vi "FWHM-TIME.vi"() -> ()   [LabVIEW 2014]
doc: "André Romero - 2017\nandretec@ifsc.usp.br"
uses:
  <vilib>/Utility/file.llb/Write To Spreadsheet File (DBL).vi
panel:
  out "Seconds":i32
  in  "Average":i32=1
  out "Waveform Graph":dbl[](graph)
  out "FWHM":dbl=7.6633162264068915
  in  "stop":bool
  out "XY Graph":T1(graph)
  in  "Correct Electrical Dark":bool=TRUE
  in  "Integration Time (ms)":i32=100
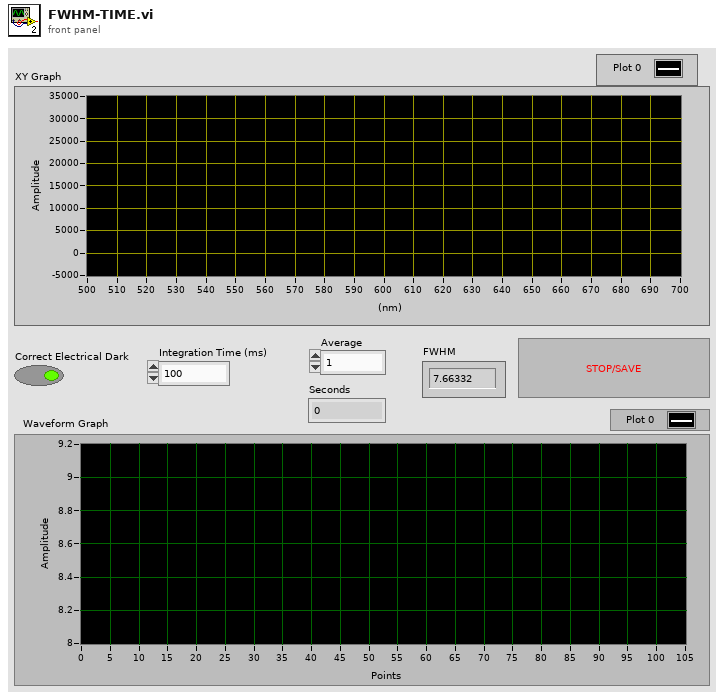
[diagram p1: front panel]
types:
  T1 = cluster{"WL Values":dbl[], "Spectrum Values":dbl[]}
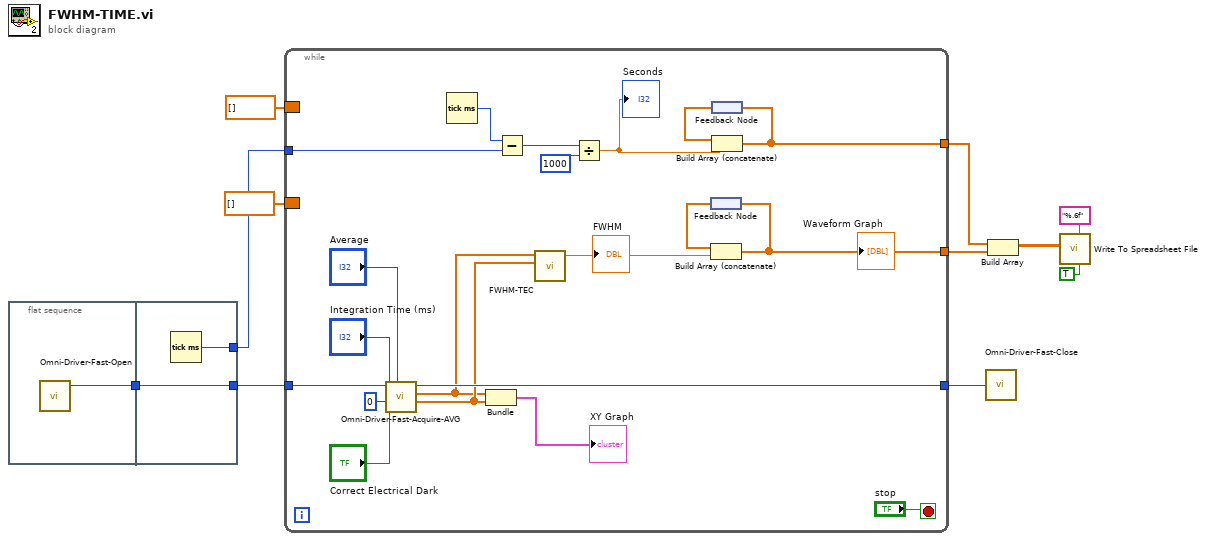
[diagram p0: block diagram]
diagram:
  n1 = flat-sequence {
    tunnel: [w12] -> w2
    tunnel: [w14] -> w11
    tunnel: w2 -> [w14]
    tunnel: [w13] -> w1
    frame #0 {
      n2 = call "Omni-Driver-Fast-Open.vi"() -> ("Wrapper Out"=w12:u32)  [unwired: 4 in, 1 out]
    }
    frame #1 {
      n3 = Tick Count (ms)() -> (millisecond timer value=w13:u32)
    }
  }
  n4 = while {
    tunnel: w11 -> [w34]
    tunnel: [w33] -> w10
    border: dbl[] [] -> [_]
    tunnel: w1 -> [w20]
    border: dbl[] [] -> [_]
    tunnel: [w18] -> w7
    tunnel: [w17] -> w6
    stop <- "stop" stop-if-true
    n5 = call "Omni-Driver-Fast-Acquire-AVG.vi"("Average"="Average", "Correct Electrical Dark"="Correct Electrical Dark", "Spectrometer number"=0, "Integration Time (ms)"="Integration Time (ms)", "Wrapper"=w34) -> ("Spectrum Values"=w27:dbl[], "WL Values"=w26:dbl[], "Wrapper Out"=w33:u32)  [unwired: 1 out]
    n6 = Tick Count (ms)() -> (millisecond timer value=w21:u32)
    n7 = Bundle("WL Values"=w26, "Spectrum Values"=w27) -> (→"XY Graph":T1)  [unwired: 1 in]
    n8 = Subtract(x=w21, y=w20) -> (x-y=w19:u32)
    n9 = call "FWHM-TEC.vi"("Y values"=w27, "WL values"=w26) -> ("FWHM"=w23:dbl)  [unwired: 9 in]
    "FWHM" <- w23
    n10 = Divide(x=w19, y=u32 1000 ("x")) -> (x/y=w15:dbl)
    "Seconds" <- w15
    n11 = feedback #1() -> (w24:dbl[])
    n12 = Build Array (concatenate)(w24, w23) -> (w17:dbl[])
    "Waveform Graph" <- w17
    n13 = feedback-in #1(w17) -> ()
    n14 = feedback #2() -> (w22:dbl[])
    n15 = Build Array (concatenate)(w22, w15) -> (w18:dbl[])
    n16 = feedback-in #2(w18) -> ()
  }
  n17 = call "Omni-Driver-Fast-Close.vi"("Wrapper In"=w10) -> ()  [unwired: 1 in]
  n18 = Build Array(w7, w6) -> (w5:dbl[][])
  n19 = call-poly <vilib>:"Write To Spreadsheet File.vi"("transpose? (no:F)"=TRUE, "format (%.3f)"="%.6f", "2D data"=w5) -> ()  [unwired: 5 in, 1 out]
